vi "Select Next Active Tab.vi"(8 "error in":errorcluster, 10 "Current Tab":i32, 11 "Tab Pages References In":refnum<vi>[](array[refnum])) -> (0 "error out":errorcluster, 2 "Next Tab":i32, 3 "Tab Pages References Out":refnum<vi>[](array[refnum]))   [LabVIEW 2017, in "DTacq Plot Display Library.lvlib"]
uses:
  DTacq Plot Display Library.lvlib
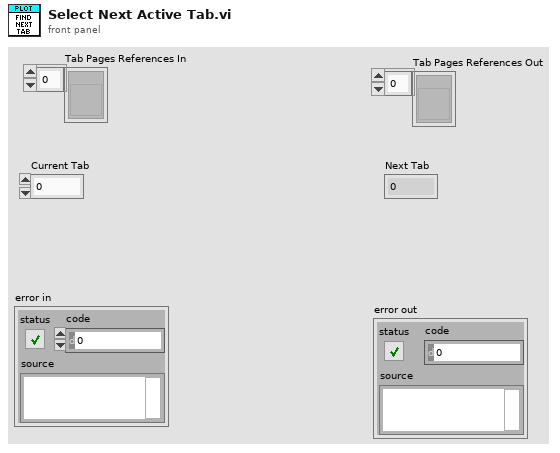
[diagram p1: front panel]
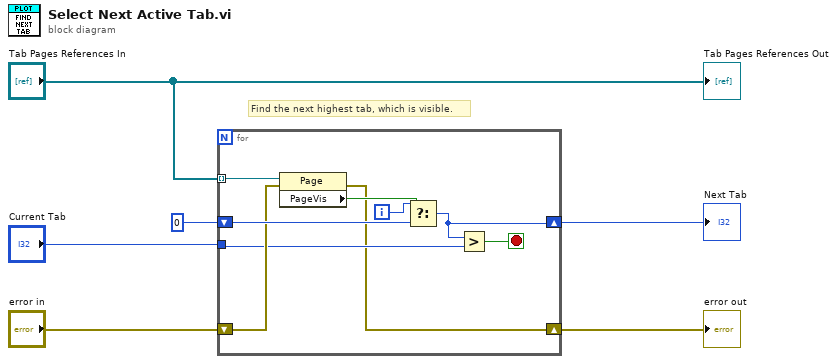
[diagram p0: block diagram]
diagram:
  # "Find the next highest tab, which is visible."
  n1 = for {
    tunnel: "Tab Pages References In" -> [w15] mode=indexing
    shift-right: [w7] -> w2
    shift-left: "error in" -> [w11]
    tunnel: "Current Tab" -> [w9]
    shift-right: [w10] -> w3
    shift-left: 0 -> [w12]
    i -> [w13]
    stop <- w8 stop-if-true
    n2 = property class="Page"(reference=w15, error in=w11) -> (error out=w7:errorcluster, "PageVis"=w14:bool)  [unwired: 1 out]
    n3 = Select(t=w13, s=w14, f=w12) -> (s? t:f=w10:i32)
    n4 = Greater?(x=w10, y=w9) -> (0:w8:bool)
  }
  "Next Tab" <- w3
  "error out" <- w2
  "Tab Pages References Out" <- "Tab Pages References In"
